vi "Execution_Appli_BuildINIFileAccToAppSettingsCluster.vi"(8 "error in":errorcluster, 10 "GenericSettings":T1, 11 "INI Path":path) -> (0 "error out":errorcluster)   [LabVIEW 2013, in "EVE.lvclass"]
uses:
  EVE.lvclass
  App_GenericSettings.ctl
  <vilib>/Utility/config.llb/Write Key (Boolean).vi
  <vilib>/Utility/config.llb/Write Key (Path).vi
  <vilib>/Utility/config.llb/Write Key (String).vi
  <vilib>/Utility/config.llb/Write Key (Double).vi
  <vilib>/Utility/config.llb/Write Key (I32).vi
  <vilib>/Utility/config.llb/NI_LVConfig.lvlib
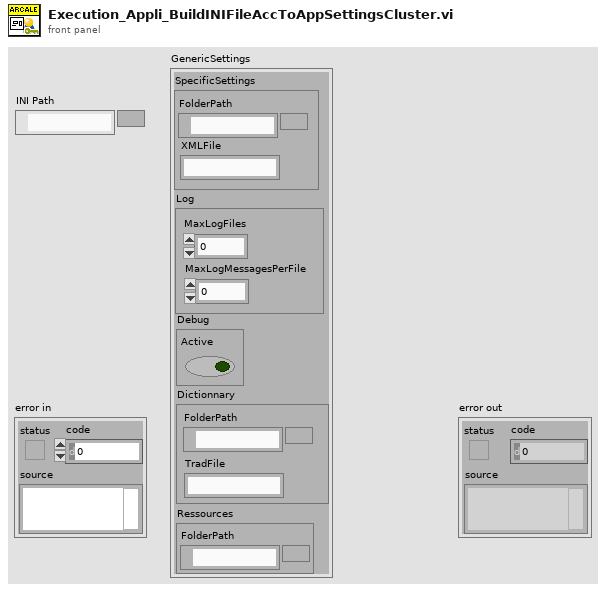
[diagram p1: front panel]
types:
  T1 = typedef "EVE.lvclass/App_GenericSettings.ctl" = cluster{"SpecificSettings":cluster{"FolderPath":path, "XMLFile":string}, "Log":cluster{"MaxLogFiles":i32, "MaxLogMessagesPerFile":i32}, "Debug":cluster{"Active":bool}, "Dictionnary":cluster{"FolderPath":path, "TradFile":string}, "Ressources":cluster{"FolderPath":path}}
  T2 = typedef "NI_LVConfig.lvlib/Config Data RefNum.ctl" = refnum<k1>
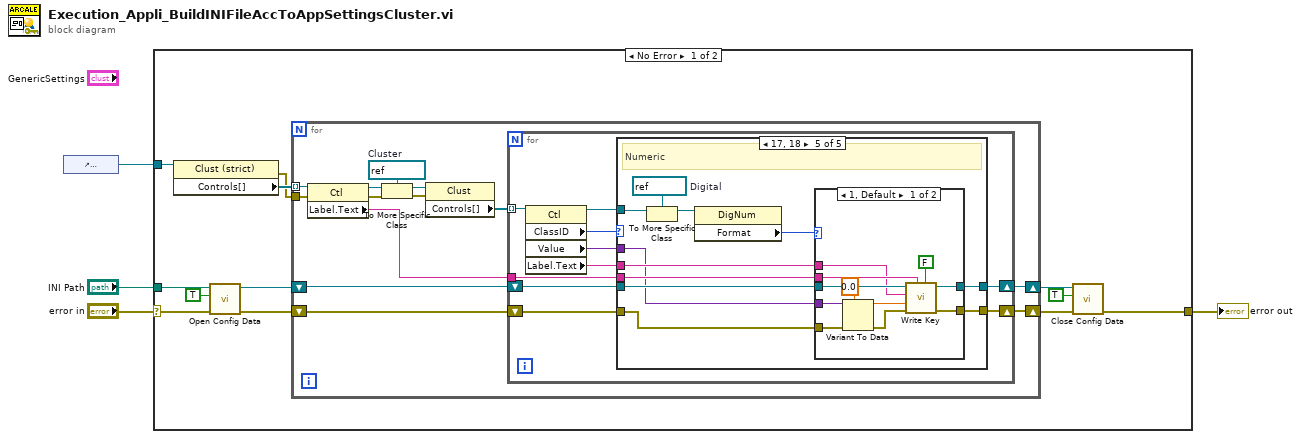
[diagram p0: block diagram]
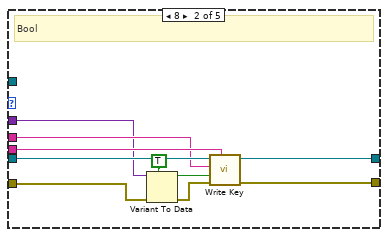
[diagram p3: hidden frame]
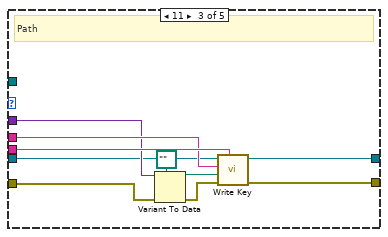
[diagram p4: hidden frame]
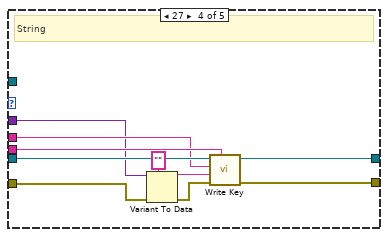
[diagram p5: hidden frame]
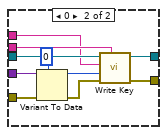
[diagram p6: hidden frame]
diagram:
  n1 = control-ref of="GenericSettings"() -> (w2:refnum<vi>)
  n2 = case shown="No Error" "error in" {
    selector: "error in" -> [w14 w104]
    tunnel: [w7 w104] -> w3
    tunnel: w2 -> [w16 _]
    tunnel: "INI Path" -> [w13 _]
    frame No Error {
      n3 = property class="Clust (strict)"(reference=w16) -> (error out=w9:errorcluster, "Controls[]"=w15:refnum<vi>[])  [unwired: 1 in, 1 out]
      n4 = call <vilib>:"Open Config Data.vi"("error in (no error)"=w14, "create file if necessary (T)"=TRUE, "configuration file path"=w13) -> ("error out"=w10:errorcluster, "refnum"=w11:T2)  [unwired: 6 in, 1 out]
      n5 = for {
        tunnel: w15 -> [w27] mode=indexing
        shift-right: [w18] -> w8
        shift-left: w10 -> [w29]
        tunnel: w9 -> [w20]
        shift-right: [w17] -> w6
        shift-left: w11 -> [w28]
        w24 = refnum<vi> refnum  # Cluster
        n6 = property class="Ctl"(reference=w27, error in=w20) -> (reference out=w26:refnum<vi>, error out=w21:errorcluster, "Label.Text"=w25:string)
        n7 = To More Specific Class(target class=w24, reference=w26, error in=w21) -> (specific class reference=w23:refnum<vi>, error out=w22:errorcluster)
        n8 = property class="Clust"(reference=w23, error in=w22) -> ("Controls[]"=w19:refnum<vi>[])  [unwired: 2 out]
        n9 = for {
          tunnel: w25 -> [w37]
          tunnel: w19 -> [w36] mode=indexing
          shift-right: [w32] -> w18
          shift-left: w29 -> [w39]
          shift-right: [w30] -> w17
          shift-left: w28 -> [w38]
          n10 = property class="Ctl"(reference=w36) -> (reference out=w31:refnum<vi>, "ClassID"=w34:u32, "Value"=w33:variant, "Label.Text"=w35:string)  [unwired: 1 in, 1 out]
          n11 = case shown="17, 18" w34 {
            tunnel: w39 -> [w41 w48 w59 w68 w79]
            tunnel: w38 -> [w40 w51 w54 w71 w82]
            tunnel: w37 -> [_ w50 w61 w70 w81]
            tunnel: w35 -> [_ w49 w60 w69 w80]
            tunnel: w33 -> [_ w46 w57 w66 w78]
            tunnel: [w41 w43 w56 w65 w77] -> w32
            tunnel: w31 -> [_ _ _ _ w76]
            tunnel: [w40 w42 w53 w63 w72] -> w30
            frame 0, Default {
            }
            frame 8 {
              # "Bool"
              n12 = Variant To Data(error in=w48, type=TRUE, Variant=w46) -> (data=w44:bool, error out=w47:errorcluster)
              n13 = call-poly <vilib>:"Write Key.vi"("section"=w50, "error in (no error)"=w47, "value"=w44, "key"=w49, "refnum"=w51) -> ("error out"=w43:errorcluster, "refnum out"=w42:T2)  [unwired: 4 in, 1 out]
            }
            frame 11 {
              # "Path"
              n14 = Variant To Data(error in=w59, type=path "", Variant=w57) -> (data=w52:path, error out=w58:errorcluster)
              n15 = call-poly <vilib>:"Write Key.vi"("section"=w61, "error in (no error)"=w58, "value"=w52, "key"=w60, "refnum"=w54) -> ("error out"=w56:errorcluster, "refnum out"=w53:T2)  [unwired: 4 in, 1 out]
            }
            frame 27 {
              # "String"
              n16 = Variant To Data(error in=w68, type="", Variant=w66) -> (data=w62:string, error out=w67:errorcluster)
              n17 = call-poly <vilib>:"Write Key.vi"("section"=w70, "error in (no error)"=w67, "value"=w62, "key"=w69, "refnum"=w71) -> ("error out"=w65:errorcluster, "refnum out"=w63:T2)  [unwired: 4 in, 1 out]
            }
            frame 17, 18 {
              w74 = refnum<vi> refnum  # Digital
              # "Numeric"
              n18 = To More Specific Class(target class=w74, reference=w76) -> (specific class reference=w75:refnum<vi>)  [unwired: 1 in, 1 out]
              n19 = property class="DigNum"(reference=w75) -> ("Format"=w73:u8)  [unwired: 1 in, 2 out]
              n20 = case shown="1, Default" w73 {
                tunnel: w82 -> [w93 w103]
                tunnel: w81 -> [w92 w102]
                tunnel: w80 -> [w91 w101]
                tunnel: w79 -> [w90 w100]
                tunnel: w78 -> [w88 w98]
                tunnel: [w87 w97] -> w77
                tunnel: [w84 w94] -> w72
                frame 1, Default {
                  n21 = Variant To Data(error in=w90, type=0.0, Variant=w88) -> (data=w85:dbl, error out=w89:errorcluster)
                  n22 = call-poly <vilib>:"Write Key.vi"("use system decimal point (T)"=FALSE, "section"=w92, "error in (no error)"=w89, "value"=w85, "key"=w91, "refnum"=w93) -> ("error out"=w87:errorcluster, "refnum out"=w84:T2)  [unwired: 3 in, 1 out]
                }
                frame 0 {
                  n23 = Variant To Data(error in=w100, type=0, Variant=w98) -> (data=w95:i32, error out=w99:errorcluster)
                  n24 = call-poly <vilib>:"Write Key.vi"("section"=w102, "error in (no error)"=w99, "value"=w95, "key"=w101, "refnum"=w103) -> ("error out"=w97:errorcluster, "refnum out"=w94:T2)  [unwired: 4 in, 1 out]
                }
              }
            }
          }
        }
      }
      n25 = call <vilib>:"Close Config Data.vi"("error in (no error)"=w8, "write file if changed (T)"=TRUE, "refnum"=w6) -> ("error out"=w7:errorcluster)  [unwired: 7 in, 1 out]
    }
    frame Error {
    }
  }
  "error out" <- w3
